vi "Write Instance.vi"(8 "error in (no error)":errorcluster, 10 "SMO.lvclass":refnum<class "SMO.lvclass">, 11 "Dependency in":refnum<class "Dependency.lvclass">) -> (0 "error out":errorcluster, 3 "Dependency out":refnum<class "Dependency.lvclass">)   [LabVIEW 2013, in "Dependency.lvclass"]
uses:
  Dependency.lvclass
  SMO/SMO.lvclass
  Dependency.lvclass/Dependency.ctl
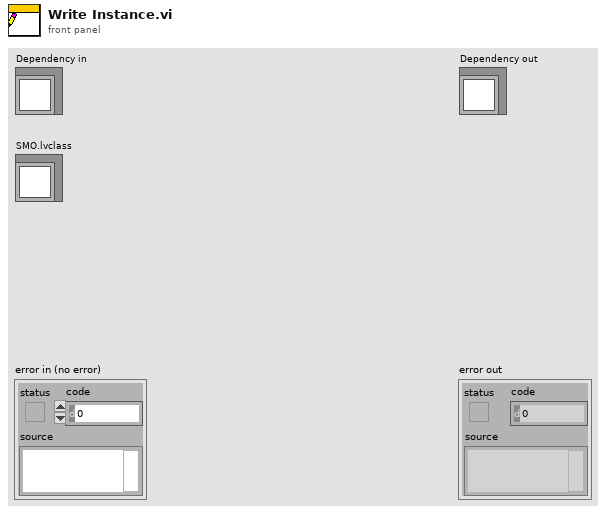
[diagram p1: front panel]
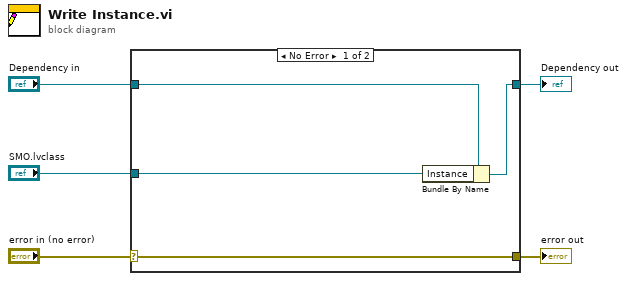
[diagram p0: block diagram]
diagram:
  n1 = case shown="No Error" "error in (no error)" {
    selector: "error in (no error)" -> [w9 w10]
    tunnel: [w9 w10] -> w4
    tunnel: [w7 w11] -> w2
    tunnel: "Dependency in" -> [w8 w11]
    tunnel: "SMO.lvclass" -> [w6 _]
    frame No Error {
      n2 = Bundle By Name(cluster=w8, "Instance"=w6) -> (w7:refnum<class "Dependency.lvclass">)
    }
    frame Error {
    }
  }
  "error out" <- w4
  "Dependency out" <- w2
